vi "oa_Build Colormap Data Output.vi"(4 "windows info":cluster{"window type":u32, "window length":i32}={"window type"=62, "window length"=2048} {"window length" min=2; "window type" items=["None"=0, "Hanning"=1, "Hamming"=2, "Blackman-Harris"=3, "Exact Blackman"=4, "Blackman"=5, "Flat Top"=6, "4 Term B-Harris"=7, "7 Term B-Harris"=8, "Low Sidelobe"=9, "Gaussian"=62]}, 5 "reset? (F)":bool, 6 "plot type":T11(ring), 7 "dB on":bool, 8 "speed profile":T7 {"speed [RPM]" format="%.2f"; "time [s]" format="%.2f"}, 9 "channel info":T8={"sensor sensitivity"=1000.0, "engineering units"=1, "dB reference"=1.0, "custom label"="EU", "weighting filter"=0, "pregain"=0.0} {"pregain" format="%.2f"; "weighting filter" items=["Linear", "A-weighting", "B-weighting", "C-weighting", "ITU-R 468-4", "Dolby", "CCITT", "C-message", "Wb", "Wc", "Wd", "We", "Wf", "Wh", "Wj", "Wk", "Wm", "AES17 20 kHz lowpass", "AES17 40 kHz lowpass", "AES17 20 kHz highpass", "AES17 40 kHz highpass"]; "dB reference" format="%^.1e"; "engineering units" items=["custom..."=0, "V"=1, "A"=21, "C"=30, "pC"=31, "s"=32, "-"=29, "Pa"=2, "N"=20, "g"=3, "m/s^2"=4, "m/s"=5, "m"=6, "mm/s"=12, "mm"=13, "micron/s"=14, "micron"=15, "in/s^2"=7, "in/s"=8, "in"=9, "mil/s"=10, "mil"=11, "rad/s^2"=16, "rad/s"=17, "rad"=18, "deg/s^2"=26, "deg/s"=27, "deg"=28, "RPM"=22, "cycle/s^2"=23, "Hz"=24, "cycle"=25, "strain"=19]; "sensor sensitivity" format="%#_5f"}, 10 "scales":T12 {"Y scale"."multiplier" format="%.2f"; "Y scale"."offset" format="%.2f"; "X scale"."multiplier" format="%.2f"; "X scale"."offset" format="%.2f"}, 11 "spectral map":dbl[][](array[numeric]) format="%.2f") -> (0 "spectrum info out":T1={"channel name"="", "description"="", "x-axis units"=0, "spectral info"={"spectrum type"=enum."Power [Magnitude^2]", "linear/dB"=enum."linear", "window"=0, "window size"=0, "FFT size"=0}, "engineering units"=0, "custom label"="", "dB reference [EU]"=0.0, "peak units"=enum."rms", "weighting filter"=0, "spectral density?"=FALSE, "unit label"="", "spectrum skewed?"=FALSE, "complimentary spectrum units"=enum."none"} {"x-axis units" items=["Time (s)"=0, "Frequency-CB (Hz)"=1, "Frequency-CPB (Hz)"=1248, "Frequency-Arbitrary (Hz)"=2357, "Quefrency (s)"=2, "Revolutions (rev)"=3, "Order"=4, "Speed (RPM)"=11, "Speed (rad/s)"=21, "Index"=65535]; "weighting filter" items=["Linear", "A-weighting", "B-weighting", "C-weighting", "ITU-R 468-4", "Dolby", "CCITT", "C-message", "Wb", "Wc", "Wd", "We", "Wf", "Wh", "Wj", "Wk", "Wm", "AES17 20 kHz lowpass", "AES17 40 kHz lowpass", "AES17 20 kHz highpass", "AES17 40 kHz highpass"]; "dB reference [EU]" format="%.2f"; "engineering units" items=["custom..."=0, "V"=1, "A"=21, "C"=30, "pC"=31, "s"=32, "-"=29, "Pa"=2, "N"=20, "g"=3, "m/s^2"=4, "m/s"=5, "m"=6, "mm/s"=12, "mm"=13, "micron/s"=14, "micron"=15, "in/s^2"=7, "in/s"=8, "in"=9, "mil/s"=10, "mil"=11, "rad/s^2"=16, "rad/s"=17, "rad"=18, "deg/s^2"=26, "deg/s"=27, "deg"=28, "RPM"=22, "cycle/s^2"=23, "Hz"=24, "cycle"=25, "strain"=19]; "spectral info"."window" items=["None "=0, "Hanning"=1, "Hamming"=2, "Blackman-Harris"=3, "Exact Blackman"=4, "Blackman"=5, "Flat Top"=6, "4 Term B-Harris "=7, "7 Term B-Harris"=8, "Low Sidelobe"=9, "Force - Exponential"=10, "Gaussian"=62]}, 1 "colormap unit labels":T9, 3 "colormap":T10 {"Y scale"."multiplier" format="%.2f"; "Y scale"."offset" format="%.2f"; "X scale"."multiplier" format="%.2f"; "X scale"."offset" format="%.2f"; "spectral map" format="%.2f"})   [LabVIEW 2017, in "SoundVib_Resampling.lvlib"]
uses:
  <vilib>/addons/Sound and Vibration/Order Analysis/Resample Order Tracking/SoundVib_Resampling.lvlib
  <vilib>/addons/_NISVFA/_Shared subVIs/Controls/svc_Channel Info.ctl
  <vilib>/addons/_NISVFA/_Shared subVIs/Controls/svc_Engineering Units Text Ring.ctl
  <vilib>/addons/_NISVFA/_Shared subVIs/Controls/svc_Weighting Filter Text Ring.ctl
  <vilib>/addons/Sound and Vibration/Order Analysis/Tach Process/SubVIs/speed profile.ctl
  <vilib>/addons/_NISVFA/_Shared subVIs/Controls/svc_Spectrum Info.ctl
  <vilib>/addons/_NISVFA/_Shared subVIs/Controls/svc_X-Axis Units.ctl
  <vilib>/addons/_NISVFA/_Shared subVIs/Controls/svc_Spectrum Type.ctl
  <vilib>/addons/_NISVFA/_Shared subVIs/Controls/svc_Complimentary Spectrum Units.ctl
  <vilib>/addons/Sound and Vibration/Order Analysis/Tach Process/SoundVib_TachProcess.lvlib
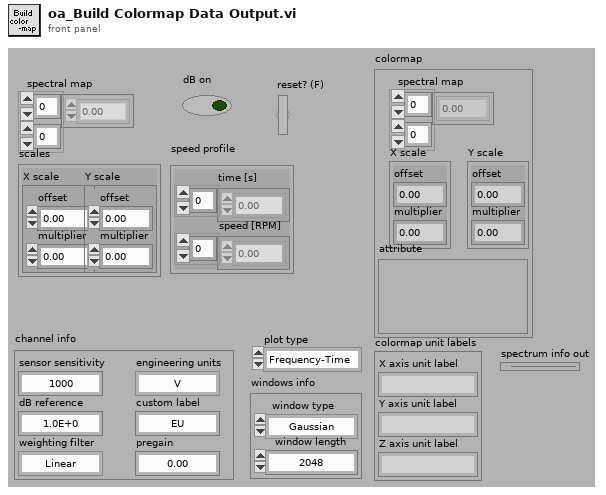
[diagram p1: front panel]
types:
  T1 = typedef "svc_Spectrum Info.ctl" = cluster{"channel name":string, "description":string, "x-axis units":T2, "spectral info":cluster{"spectrum type":T3, "linear/dB":enum16{"linear", "dB"}, "window":u16, "window size":i32, "FFT size":i32}, "engineering units":T4, "custom label":string, "dB reference [EU]":dbl, "peak units":enum16{"rms", "peak", "peak-peak"}, "weighting filter":T5, "spectral density?":bool, "unit label":string, "spectrum skewed?":bool, "complimentary spectrum units":T6}
  T2 = typedef "svc_X-Axis Units.ctl" = u16
  T3 = typedef "svc_Spectrum Type.ctl" = enum16{"FFT Spectrum [complex]", "Amplitude [Magnitude]", "Power [Magnitude^2]", "Cross Spectrum [complex]", "Frequency Response [Complex]"}
  T4 = typedef "svc_Engineering Units Text Ring.ctl" = u16
  T5 = typedef "svc_Weighting Filter Text Ring.ctl" = u16
  T6 = typedef "svc_Complimentary Spectrum Units.ctl" = enum16{"none", "radians", "degrees", "cycles", "imaginary"}
  T7 = typedef "SoundVib_TachProcess.lvlib/speed profile.ctl" = cluster{"time [s]":dbl[], "speed [RPM]":dbl[]}
  T8 = typedef "svc_Channel Info.ctl" = cluster{"sensor sensitivity":dbl, "engineering units":T4, "dB reference":dbl, "custom label":string, "weighting filter":T5, "pregain":dbl}
  T9 = cluster{"X axis unit label":string, "Y axis unit label":string, "Z axis unit label":string}
  T10 = cluster{"spectral map":dbl[][], "X scale":cluster{"offset":dbl, "multiplier":dbl}, "Y scale":cluster{"offset":dbl, "multiplier":dbl}, "attribute":variant}
  T11 = enum16{"Frequency-Time", "Time-Frequency", "Order-Time", "Time-Order", "Frequency-RPM", "RPM-Frequency", "Order-RPM", "RPM-Order"}
  T12 = cluster{"X scale":cluster{"offset":dbl, "multiplier":dbl}, "Y scale":cluster{"offset":dbl, "multiplier":dbl}}
  T13 = cluster{"log view scaled signal":dbl[][], "Y scale":cluster{"offset":dbl, "multiplier":dbl}, "X scale":cluster{"offset":dbl, "multiplier":dbl}, "variant":variant}
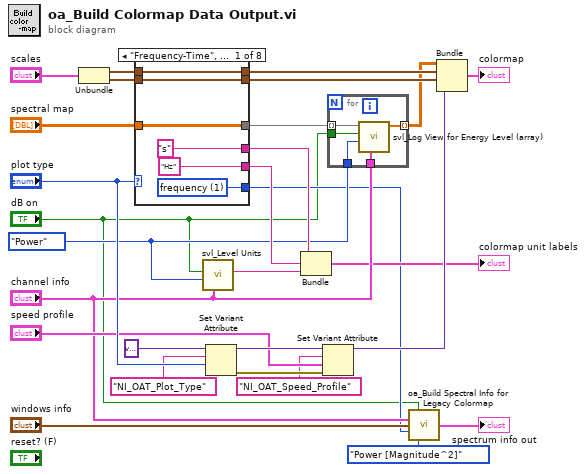
[diagram p0: block diagram]
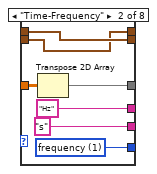
[diagram p2: hidden frame]
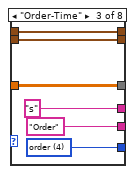
[diagram p3: hidden frame]
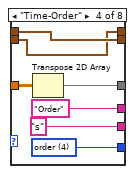
[diagram p4: hidden frame]
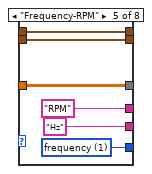
[diagram p5: hidden frame]
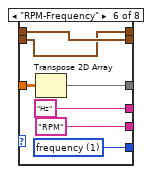
[diagram p6: hidden frame]
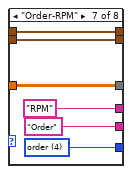
[diagram p7: hidden frame]
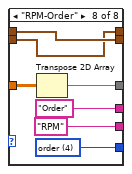
[diagram p8: hidden frame]
diagram:
  w3 = enum16{"Power", "Amplitude"}."Power" ("view mode")
  n1 = Unbundle("scales") -> ("X scale"=w26:cluster{"offset":dbl, "multiplier":dbl}, "Y scale"=w25:cluster{"offset":dbl, "multiplier":dbl})
  n2 = case shown="\"Frequency-Time\", Default" "plot type" {
    tunnel: "spectral map" -> [w31 w41 w44 w54 w57 w67 w70 w80]
    tunnel: w26 -> [w34 w40 w47 w53 w60 w66 w73 w79]
    tunnel: w25 -> [w33 w35 w46 w48 w59 w65 w72 w78]
    tunnel: [w31 w38 w44 w51 w57 w63 w70 w76] -> w10
    tunnel: [w34 w35 w47 w48 w60 w65 w73 w78] -> w17
    tunnel: [w33 w40 w46 w53 w59 w66 w72 w79] -> w16
    tunnel: [w32 w39 w45 w52 w58 w64 w71 w77] -> w2
    tunnel: ["s" "Hz" "s" "Order" "RPM" "Hz" "RPM" "Order"] -> w8
    tunnel: ["Hz" "s" "Order" "s" "Hz" "RPM" "Order" "RPM"] -> w7
    frame "Frequency-Time", Default {
      w32 = u16 1 items=["time"=0, "frequency"=1, "quefrency"=2, "revolutions"=3, "order"=4, "rpm"=11] ("x-axis units")
    }
    frame "Time-Frequency" {
      w39 = u16 1 items=["time"=0, "frequency"=1, "quefrency"=2, "revolutions"=3, "order"=4, "rpm"=11] ("x-axis units")
      n3 = Transpose 2D Array(2D array=w41) -> (transposed array=w38:dbl[][])
    }
    frame "Order-Time" {
      w45 = u16 4 items=["time"=0, "frequency"=1, "quefrency"=2, "revolutions"=3, "order"=4, "rpm"=11] ("x-axis units")
    }
    frame "Time-Order" {
      w52 = u16 4 items=["time"=0, "frequency"=1, "quefrency"=2, "revolutions"=3, "order"=4, "rpm"=11] ("x-axis units")
      n4 = Transpose 2D Array(2D array=w54) -> (transposed array=w51:dbl[][])
    }
    frame "Frequency-RPM" {
      w58 = u16 1 items=["time"=0, "frequency"=1, "quefrency"=2, "revolutions"=3, "order"=4, "rpm"=11] ("x-axis units")
    }
    frame "RPM-Frequency" {
      w64 = u16 1 items=["time"=0, "frequency"=1, "quefrency"=2, "revolutions"=3, "order"=4, "rpm"=11] ("x-axis units")
      n5 = Transpose 2D Array(2D array=w67) -> (transposed array=w63:dbl[][])
    }
    frame "Order-RPM" {
      w71 = u16 4 items=["time"=0, "frequency"=1, "quefrency"=2, "revolutions"=3, "order"=4, "rpm"=11] ("x-axis units")
    }
    frame "RPM-Order" {
      w77 = u16 4 items=["time"=0, "frequency"=1, "quefrency"=2, "revolutions"=3, "order"=4, "rpm"=11] ("x-axis units")
      n6 = Transpose 2D Array(2D array=w80) -> (transposed array=w76:dbl[][])
    }
  }
  n7 = call <vilib>:"svl_Level Units.vi"("channel info"="channel info", "view mode"=w3, "dB On (T)"="dB on") -> ("unit label"=w5:string)  [unwired: 6 in, 2 out]
  n8 = Set Variant Attribute(Variant=variant ("variant"), name="NI_OAT_Plot_Type", value="plot type") -> (Variant out=w21:variant, error out=w22:errorcluster)  [unwired: 1 in, 1 out]
  n9 = Bundle(w8, w7, "unit label"=w5) -> (→"colormap unit labels":cluster{string, string, "unit label":string})  [unwired: 1 in]
  n10 = Set Variant Attribute(Variant=w21, name="NI_OAT_Speed_Profile", value="speed profile", error in=w22) -> (Variant out=w18:variant)  [unwired: 2 out]
  n11 = for {
    tunnel: [w85] -> w9 mode=indexing
    tunnel: w10 -> [w84] mode=indexing
    tunnel: "channel info" -> [w83]
    tunnel: w3 -> [w82]
    tunnel: "dB on" -> [w81]
    n12 = call <vilib>:"svl_Log View for Energy Level (array).vi"("channel info"=w83, "view mode"=w82, "dB On (T)"=w81, "scaled signal"=w84) -> ("log view scaled signal"=w85:dbl[])  [unwired: 5 in, 2 out]
  }
  n13 = call <vilib>:"oa_Build Spectral Info for Legacy Colormap.vi"("dB on (T)"="dB on", "channel info"="channel info", "windows info"="windows info", "x-axis units"=w2, "spectrum type"=svc_Spectrum_Type."Power [Magnitude^2]") -> ("spectrum info"=→"spectrum info out":T1)  [unwired: 9 in, 1 out]
  n14 = Bundle("log view scaled signal"=w9, "Y scale"=w17, "X scale"=w16, "variant"=w18) -> (→"colormap":T13)  [unwired: 1 in]
